vi "DriveEncoderToDashBoard.vi"(10 "EncoderDevRef":T1, 11 "EncoderDevRef 2":T1) -> ()   [LabVIEW 2016]
uses:
  <vilib>/Rock Robotics/WPI/Encoder/WPI_EncoderDevRef.ctl
  <vilib>/Rock Robotics/SystemInterfaces/Encoder/FPGA_EncoderIdx.ctl
  <vilib>/Rock Robotics/SystemInterfaces/Counter/FPGA_CounterCtrSystemIndex.ctl
  <vilib>/Rock Robotics/WPI/Encoder/WPI_EncoderType.ctl
  <vilib>/Rock Robotics/Network Tables/NT Write Number.vi
  <vilib>/Rock Robotics/Network Tables/NT Read Number.vi
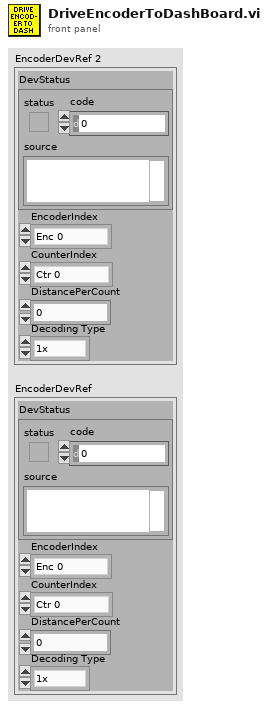
[diagram p1: front panel]
types:
  T1 = typedef "WPI_EncoderDevRef.ctl" = cluster{"DevStatus":errorcluster, "EncoderIndex":T2, "CounterIndex":T3, "DistancePerCount":dbl, "Decoding Type":T4}
  T2 = typedef "FPGA_EncoderIdx.ctl" = enum8{"Enc 0", "Enc 1", "Enc 2", "Enc 3", "Enc 4", "Enc 5", "Enc 6", "Enc 7", "Invalid"}
  T3 = typedef "FPGA_CounterCtrSystemIndex.ctl" = enum8{"Ctr 0", "Ctr 1", "Ctr 2", "Ctr 3", "Ctr 4", "Ctr 5", "Ctr 6", "Ctr 7", "Invalid"}
  T4 = typedef "WPI_EncoderType.ctl" = enum16{"1x", "2x", "4x"}
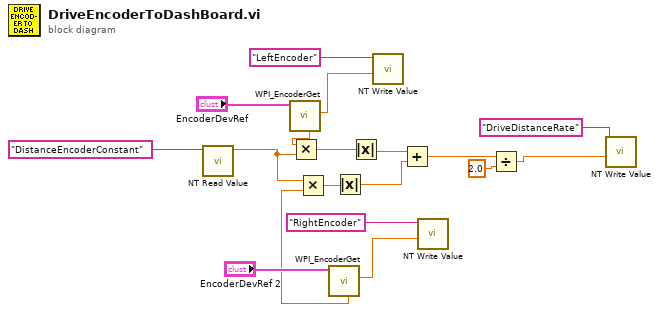
[diagram p0: block diagram]
diagram:
  n1 = call-poly <vilib>:"NT Read Value.vi"("Name"="DistanceEncoderConstant") -> ("Numeric"=w4:dbl)  [unwired: 9 in, 1 out]
  n2 = call <vilib>:"WPI_EncoderGet.vi"("EncoderDevRef"="EncoderDevRef") -> ("Distance"=w15:dbl, "Rate"=w5:dbl)  [unwired: 5 in, 4 out]
  n3 = Multiply(x=w5, y=w4) -> (x*y=w6:dbl)
  n4 = call <vilib>:"WPI_EncoderGet.vi"("EncoderDevRef"="EncoderDevRef 2") -> ("Distance"=w16:dbl, "Rate"=w3:dbl)  [unwired: 5 in, 4 out]
  n5 = Multiply(x=w4, y=w3) -> (x*y=w7:dbl)
  n6 = Absolute Value(x=w7) -> (abs(x)=w2:dbl)
  n7 = Absolute Value(x=w6) -> (abs(x)=w1:dbl)
  n8 = call-poly <vilib>:"NT Write Value.vi"("Numeric"=w15, "Name"="LeftEncoder") -> ()  [unwired: 9 in, 1 out]
  n9 = Add(x=w1, y=w2) -> (x+y=w11:dbl)
  n10 = call-poly <vilib>:"NT Write Value.vi"("Numeric"=w16, "Name"="RightEncoder") -> ()  [unwired: 9 in, 1 out]
  n11 = Divide(x=w11, y=2.0) -> (x/y=w10:dbl)
  n12 = call-poly <vilib>:"NT Write Value.vi"("Numeric"=w10, "Name"="DriveDistanceRate") -> ()  [unwired: 9 in, 1 out]
